vi "Initialize Front Panel.vi"(8 "error in (no error)":errorcluster, 11 "BoundViewManager in":refnum<class "BoundViewManager.lvclass">) -> (0 "error out":errorcluster, 3 "BoundViewManager out":refnum<class "BoundViewManager.lvclass">)   [LabVIEW 2017, in "BoundViewManager.lvlib" / "BoundViewManager.lvclass"]
doc: "<License>\nCopyright © 2017 Composed Systems, LLC | All rights reserved\nwww.composed.io\n\nAuthor: Ethan Stern <ethan.stern@composed.io>\n\nThis software is provided \"AS IS\" WITHOUT WARRANTIES, either express or implied, AND IS FOR EDUCATIONAL PURPOSES ONLY.\n</License>"
uses:
  BoundViewManager.lvclass
  <vilib>/ActorFramework/Message Enqueuer/Message Enqueuer.lvclass
  gpm_packages/@cs/mva-viewable/Source/IViewable/IViewable Messages/Insert Front Panel Msg/Insert Front Panel Msg.lvclass
  61cc6e39-6280-4a2f-9646-d72848929907.vi
  gpm_packages/@cs/mva-viewable/Source/IViewManager/IViewManager/IViewManager.lvclass
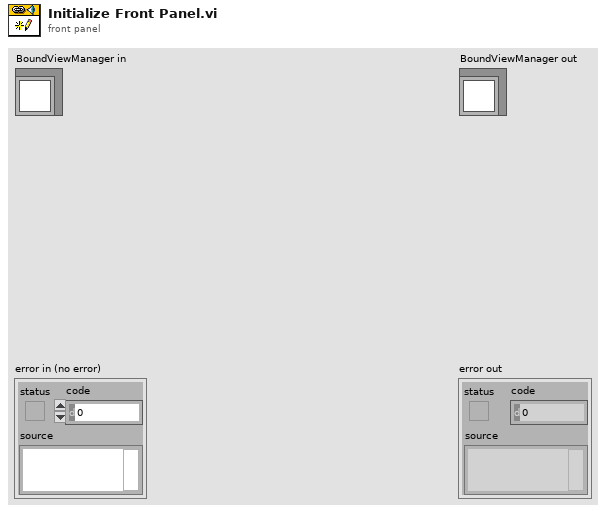
[diagram p1: front panel]
types:
  T1 = typedef "IViewable.lvlib/ProtectedSubpanel.lvclass/Protected Subpanel Reference.ctl" = refnum<data-value>
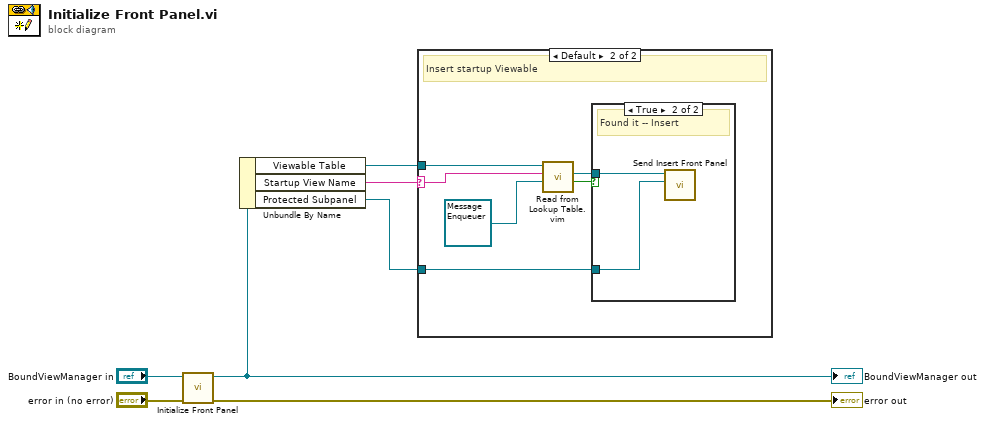
[diagram p0: block diagram]
diagram:
  n1 = call-parent "Initialize Front Panel.vi"("error in (no error)"="error in (no error)", "IViewable in"="BoundViewManager in") -> ("error out"=→"error out":errorcluster, "IViewable out"=w4:refnum<class "BoundViewManager.lvclass">)  [unwired: 8 in]
  "BoundViewManager out" <- w4
  n2 = Unbundle By Name(w4) -> ("Viewable Table"=w2:refnum<data-value>, "Startup View Name"=w3:string, "Protected Subpanel"=w1:T1)
  n3 = case shown="Default" w3 {
    selector: w3 -> [_ w12]
    tunnel: w2 -> [_ w13]
    tunnel: w1 -> [_ w9]
    frame "" {
      # "No startup viewable insertion"
    }
    frame Default {
      # "Insert startup Viewable"
      n4 = call "Read from Lookup Table.vim"("Type"=refnum<class "Message Enqueuer.lvclass"> refnum ("Message Enqueuer"), "Item Name"=w12, "LookupTable Reference"=w13) -> ("Not Found?"=w11:bool, "Value"=w10:refnum<class "Message Enqueuer.lvclass">)  [unwired: 5 in, 2 out]
      n5 = case shown="True" w11 {
        tunnel: w10 -> [_ w14]
        tunnel: w9 -> [_ w15]
        frame False {
          # "Not found"
        }
        frame True {
          # "Found it -- Insert"
          n6 = call "Send Insert Front Panel.vi"("Protected Subpanel"=w15, "Message Enqueuer"=w14) -> ()  [unwired: 8 in, 2 out]
        }
      }
    }
  }
